vi "get channel info.vi"(1 "device type":T2=enum."LAN") -> (0 "device channel spec":T1={"upper channel limit"=1, "lower channel limit"=1, "channel base"=0} {"channel base" format="%x"})   [LabVIEW 2024, in "atsj peakcan basic.lvlib"]
doc: "Gets channel information for a specific device type."
uses:
  atsj peakcan basic.lvlib
  device type.ctl
  channel info.ctl
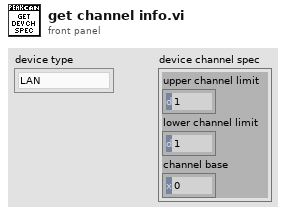
[diagram p1: front panel]
types:
  T1 = typedef "atsj peakcan basic.lvlib/channel info.ctl" = cluster{"upper channel limit":u8, "lower channel limit":u8, "channel base":u16}
  T2 = typedef "atsj peakcan basic.lvlib/device type.ctl" = enum8{"ISA", "DNG", "PCI", "USB", "PCC", "LAN"}
  T3 = cluster{"upper channel limit":u8, "lower channel limit":u8, "channel base":u16}[]
  T4 = cluster{"upper channel limit":u8, "lower channel limit":u8, "channel base":u16}
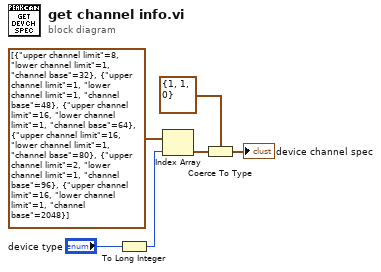
[diagram p0: block diagram]
diagram:
  n1 = To Long Integer(number="device type") -> (32bit integer=w4:i32)
  n2 = Index Array(array=T3 [{"upper channel limit"=8, "lower channel limit"=1, "channel base"=32}, {"upper channel limit"=1, "lower channel limit"=1, "channel base"=48}, {"upper channel limit"=16, "lower channel limit"=1, "channel base"=64}, {"upper channel limit"=16, "lower channel limit"=1, "channel base"=80}, {"upper channel limit"=2, "lower channel limit"=1, "channel base"=96}, {"upper channel limit"=16, "lower channel limit"=1, "channel base"=2048}], index=w4) -> (element=w3:T4)
  n3 = Coerce To Type(0:w3, 1:T1 {"upper channel limit"=1, "lower channel limit"=1, "channel base"=0}) -> (2:→"device channel spec":T1)
